vi "Get Operating Mode.vi"(8 "error in (no error)":errorcluster, 11 "Item Ref in":T2 format="%.0x") -> (0 "error out":errorcluster, 2 "Operating mode":T1=enum."Single Stepping", 3 "Item Ref out":T2 format="%.0x")   [LabVIEW 2019, in "TimingDRV System Explorer.lvlib"]
uses:
  TimingDRV System Explorer.lvlib
  <vilib>/NI VeriStand/Custom Device API/Custom Device Item Ref.ctl
  TypeDefs/Operating Mode Types.ctl
  Engine/Parent Classes/Process/Process.lvclass
  Engine/Processes/Single Stepped TS/STS Process.lvclass
  C:/Users/XEnderMD/Desktop/CD Project Tools/Source/Engine/Parent Classes/Process/Process.lvclass
  Engine/Processes/TCP Process/TCP Process.lvclass
  Engine/Processes/Free Running TS/FRTS Process.lvclass
  <vilib>/NI VeriStand/Custom Device API/Get Item Property (String).vi
  <vilib>/NI VeriStand/Custom Device API/Custom Device API.lvlib
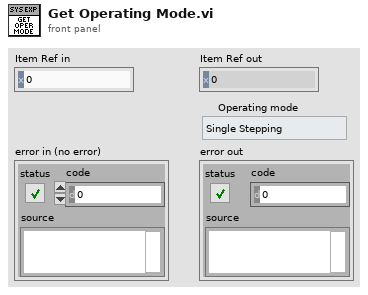
[diagram p1: front panel]
types:
  T1 = typedef "TimingDRV System Explorer.lvlib/Operating Mode Types.ctl" = enum16{"Free Running", "Single Stepping"}
  T2 = typedef "Custom Device API.lvlib/Custom Device Item Ref.ctl" = u64
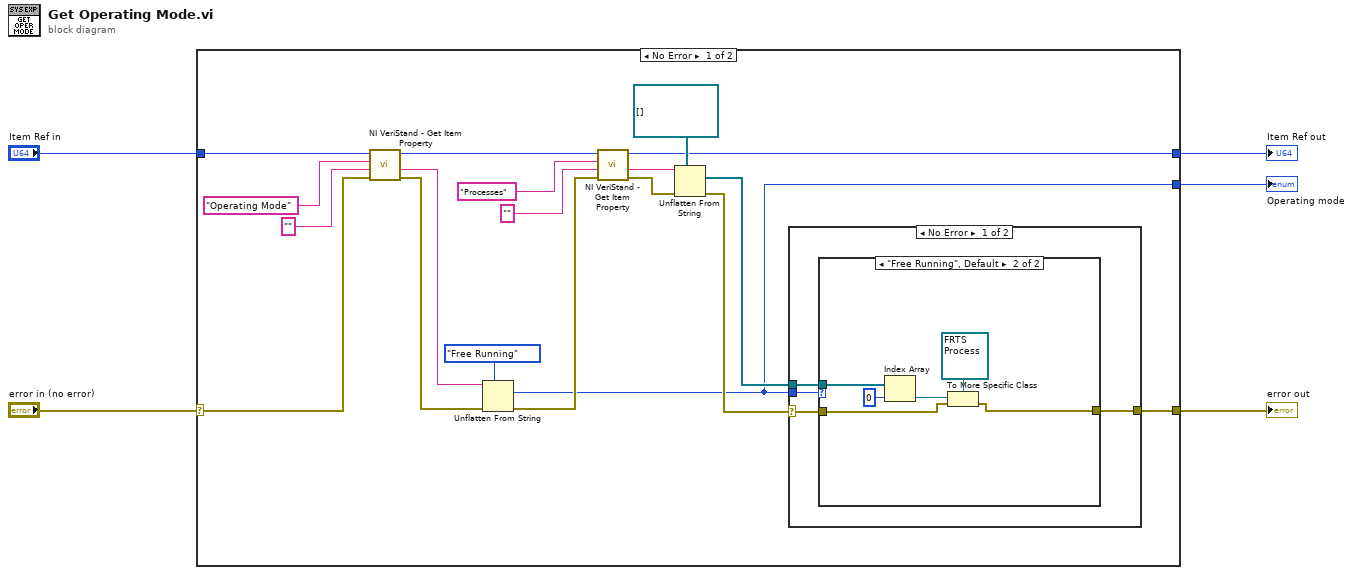
[diagram p0: block diagram]
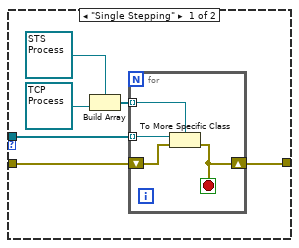
[diagram p2: hidden frame]
diagram:
  n1 = case shown="No Error" "error in (no error)" {
    selector: "error in (no error)" -> [w9 w47]
    tunnel: "Item Ref in" -> [w21 w46]
    tunnel: [w8 w47] -> w3
    tunnel: [w7 w46] -> w2
    tunnel: [w6 _] -> w1
    frame No Error {
      n2 = call-poly <vilib>:"NI VeriStand - Get Item Property.vi"("error in (no error)"=w9, "Default Value"="", "Property Name"="Operating Mode", "Item Ref in"=w21) -> ("error out"=w24:errorcluster, "Value"=w23:string, "Item Ref out"=w17:T2)  [unwired: 4 in, 1 out]
      n3 = Unflatten From String(type=Operating_Mode_Types."Free Running" ("Operating mode"), binary string=w23, error in (no error)=w24) -> (value=w6:T1, error out=w18:errorcluster)  [unwired: 2 in, 1 out]
      n4 = call-poly <vilib>:"NI VeriStand - Get Item Property.vi"("error in (no error)"=w18, "Default Value"="", "Property Name"="Processes", "Item Ref in"=w17) -> ("error out"=w12:errorcluster, "Value"=w14:string, "Item Ref out"=w7:T2)  [unwired: 4 in, 1 out]
      n5 = Unflatten From String(type=refnum<class "Process.lvclass">[] [], binary string=w14, error in (no error)=w12) -> (value=w10:refnum<class "Process.lvclass">[], error out=w11:errorcluster)  [unwired: 2 in, 1 out]
      n6 = case shown="No Error" w11 {
        selector: w11 -> [w26 w45]
        tunnel: w6 -> [w28 _]
        tunnel: w10 -> [w27 _]
        tunnel: [w25 w45] -> w8
        frame No Error {
          n7 = case shown="\"Free Running\", Default" w28 {
            tunnel: w27 -> [w34 w44]
            tunnel: w26 -> [w30 w40]
            tunnel: [w29 w39] -> w25
            frame "Single Stepping" {
              n8 = Build Array(refnum<class "STS Process.lvclass"> refnum ("TimingDRV Engine.lvlib:STS Process.lvclass"), refnum<class "TCP Process.lvclass"> refnum ("TimingDRV Engine.lvlib:TCP Process.lvclass")) -> (w31:refnum<class "Process.lvclass">[])
              n9 = for {
                tunnel: w34 -> [w38] mode=indexing
                tunnel: w31 -> [w37] mode=indexing
                shift-right: [w35] -> w29
                shift-left: w30 -> [w36]
                stop <- w35 stop-if-true
                n10 = To More Specific Class(target class=w37, reference=w38, error in=w36) -> (error out=w35:errorcluster)  [unwired: 1 out]
              }
            }
            frame "Free Running", Default {
              n11 = Index Array(array=w44, index=0) -> (element=w42:refnum<class "Process.lvclass">)
              n12 = To More Specific Class(target class=refnum<class "FRTS Process.lvclass"> refnum ("TimingDRV Engine.lvlib:FRTS Process.lvclass"), reference=w42, error in=w40) -> (error out=w39:errorcluster)  [unwired: 1 out]
            }
          }
        }
        frame Error {
        }
      }
    }
    frame Error {
    }
  }
  "error out" <- w3
  "Item Ref out" <- w2
  "Operating mode" <- w1
